vi "Test - Multiple Random Numbers.vi"() -> ()   [LabVIEW 2014, in "HMM.lvlib"]
uses:
  HMM.lvlib
  <vilib>/Analysis/NI_AALBase.lvlib
panel:
  in  "stop":bool
  in  "N-th value":i32
  in  "No. of rands":i32=3
  out "Histogram Graph":T1(graph)
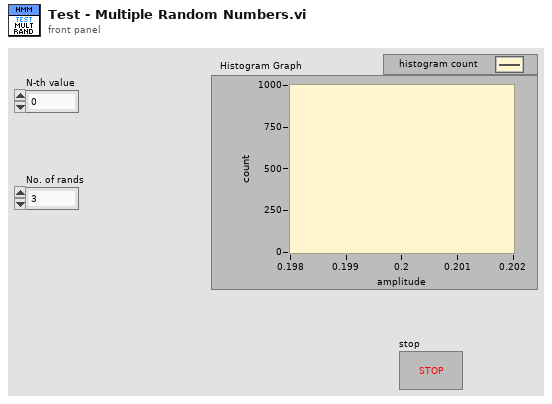
[diagram p1: front panel]
types:
  T1 = cluster{"X Values":dbl[], "Histogram: h(x)":i32[]}
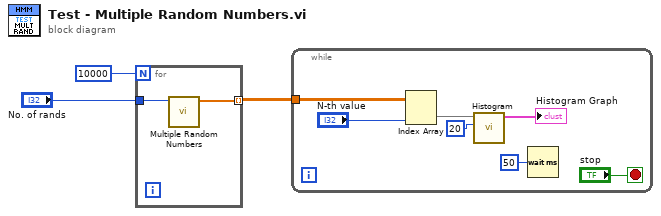
[diagram p0: block diagram]
diagram:
  n1 = for {
    N: 10000 -> [_]
    tunnel: "No. of rands" -> [w5]
    tunnel: [w4] -> w1 mode=indexing
    n2 = call "Multiple Random Numbers.vi"("No. of rands"=w5) -> ("Random numbers"=w4:dbl[])  [unwired: 10 in]
  }
  n3 = while {
    tunnel: w1 -> [w12]
    stop <- "stop" stop-if-true
    n4 = Index Array(array=w12, index (col)="N-th value") -> (element=w9:dbl[])  [unwired: 1 in]
    n5 = call <vilib>:"Histogram.vi"("intervals"=20, "X"=w9) -> ("Histogram Graph"=→"Histogram Graph":T1)  [unwired: 6 in, 3 out]
    n6 = Wait (ms)(milliseconds to wait=u32 50) -> ()  [unwired: 1 out]
  }
